vi "Teleop.vi"(10 "Match Info":T1={"Autonomous Elapsed Seconds"=0.0, "TeleOp Elapsed Seconds"=0.0, "Disabled Elapsed Seconds"=0.0, "Visited Autonomous"=FALSE, "Visited TeleOp"=FALSE, "Visited Disabled"=FALSE, "Autonomous Settings"={"Autonomous Style"=enum."Independent", "VI Refnum"=refnum}}, 11 "Call Context":T2) -> ()   [LabVIEW 2015]
doc: "This VI is called for each TeleOp packet received from the DS where the robot is not disabled. It is often used to read from the joysticks and update I/O or to update setpoints for timed control loops. It should complete and return within 20 milliseconds or it may miss DS packets."
uses:
  <vilib>/Rock Robotics/WPI/DriverStation/WPI_DriverStationDerivedRobotMode.ctl
  <vilib>/Rock Robotics/WPI/DriverStation/WPI_DriverStationMatch Info.ctl
  <vilib>/Rock Robotics/WPI/Utilities/WPI_GetSetVariantRefNum.vi
  <vilib>/Rock Robotics/Network Tables/NT Write Boolean Array.vi
  <vilib>/Rock Robotics/Network Tables/NT Write Numeric Array.vi
  <vilib>/Rock Robotics/WPI/RobotDrive/WPI_RobotDriveMecanumDrive_Cartesian.vi
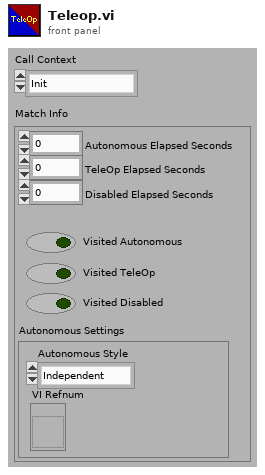
[diagram p1: front panel]
types:
  T1 = typedef "WPI_DriverStationMatch Info.ctl" = cluster{"Autonomous Elapsed Seconds":dbl, "TeleOp Elapsed Seconds":dbl, "Disabled Elapsed Seconds":dbl, "Visited Autonomous":bool, "Visited TeleOp":bool, "Visited Disabled":bool, "Autonomous Settings":cluster{"Autonomous Style":enum16{"Iterative", "Independent"}, "VI Refnum":refnum<vi>}}
  T2 = typedef "WPI_DriverStationDerivedRobotMode.ctl" = enum16{"Init", "Execute", "Stop"}
  T3 = typedef "WPI_JoystickDevRef.ctl" = cluster{"Device":T4}
  T4 = typedef "WPI_JoystickDeviceEnum.ctl" = enum16{"USB 0", "USB 1", "USB 2", "USB 3", "USB 4", "USB 5"}
  T5 = typedef "WPI_RobotDriveDevRef.ctl" = cluster{"DevStatus":errorcluster, "Motors[]":T6[], "Square Inputs":bool, "Max Output":dbl}
  T6 = typedef "WPI_MotorControlDeviceRef.ctl" = cluster{"DeviceStatus":errorcluster, "Type":T7, "PWM":cluster{"PWM Channel":T8, "DeadBand":T9}, "CAN":cluster{"Device Number":u8, "Control Mode":T10, "Semaphore":T11, "Max Vout":dbl, "TalonSRX Control Mode":T12}, "Invert":bool}
  T7 = typedef "WPI_MotorControlType.ctl" = enum16{"PWM", "CAN", "CANTalonSRX"}
  T8 = typedef "FPGA_DIOPWMChannel.ctl" = enum8{"PWM 0", "PWM 1", "PWM 2", "PWM 3", "PWM 4", "PWM 5", "PWM 6", "PWM 7", "PWM 8", "PWM 9", "PWM MXP 0", "PWM MXP 1", "PWM MXP 2", "PWM MXP 3", "PWM MXP 4", "PWM MXP 5", "PWM MXP 6", "PWM MXP 7", "PWM MXP 8", "PWM MXP 9", "Invalid"}
  T9 = typedef "WPI_PWMDeadband.ctl" = cluster{"Name":string, "maxPositivePwm":i32, "minPositivePwm":i32, "centerPwm":i32, "maxNegativePwm":i32, "minNegativePwm":i32, "angularRange":u16}
  T10 = typedef "WPI_CANJaguar_ControlMode.ctl" = enum8{"Percent VBus", "Current", "Speed", "Position", "Voltage"}
  T11 = typedef "Semaphore RefNum" = refnum<k1>
  T12 = typedef "WPI_CANTalonSRX_APIControlMode.ctl" = enum8{"Percent VBus", "Speed", "Position", "Slave", "Unchanged / Invalid", "Voltage Compensation", "Current", "Motion Profile"}
  T13 = typedef "WPI_GyroDevRef.ctl" = cluster{"DevStatus":errorcluster, "Analog Channel":T14, "Offset":dbl, "Gain (VoltsPerDegree/Second)":dbl, "Gyro Type":enum16{"Analog", "XRS450"}, "Handle":i32, "SPI Bus":T15, "Device Found":bool, "Sample Rate":dbl, "Calibrate On Open":bool}
  T14 = typedef "FPGA_AIChannel.ctl" = enum8{"AI 0", "AI 1", "AI 2", "AI 3", "AI MXP 0", "AI MXP 1", "AI MXP 2", "AI MXP 3", "Invalid"}
  T15 = typedef "spi_bus.ctl" = enum16{"SPI On-Board, CS0", "SPI On-Board, CS1", "SPI On-Board, CS2", "SPI On-Board, CS3", "SPI MXP", "Invalid"}
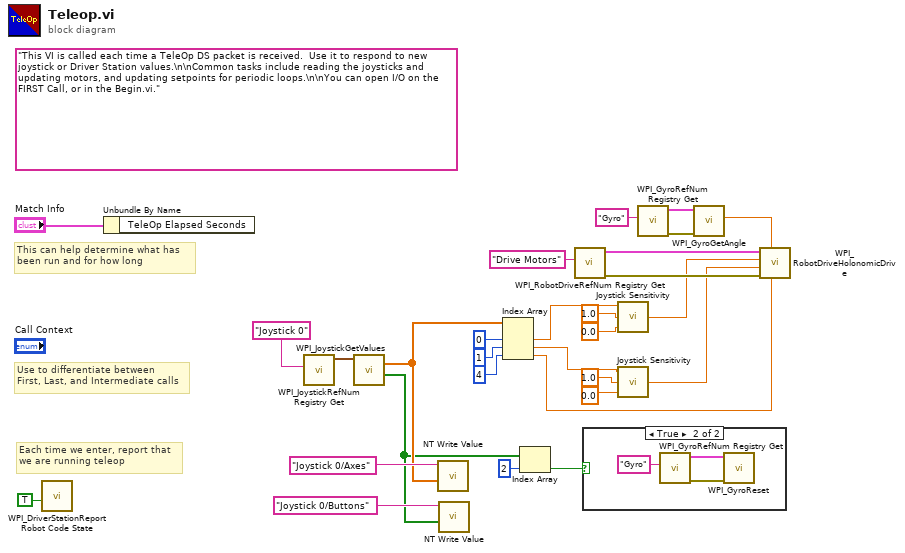
[diagram p0: block diagram]
diagram:
  (unwired) "This VI is called each time a TeleOp DS packet is received.  Use it to respond to new joystick or Driver Station values.\n\nCommon tasks include reading the joysticks and updating motors, and updating setpoints for periodic loops.\n\nYou can open I/O on the FIRST Call, or in the Begin.vi."
  # "Each time we enter, report that\nwe are running teleop"
  # "Use to differentiate between\nFirst, Last, and Intermediate calls"
  # "This can help determine what has\nbeen run and for how long"
  n1 = call <vilib>:"WPI_DriverStationReport Robot Code State.vi"("TeleOp"=TRUE ("Autonomous")) -> ()  [unwired: 10 in, 1 out]
  n2 = Unbundle By Name("Match Info") -> ()  [unwired: 1 out]
  n3 = call <vilib>:"WPI_JoystickRefNum Registry Get.vi"("refnum name"="Joystick 0") -> ("JoystickDevRef"=w24:T3)  [unwired: 1 in, 9 out]
  n4 = call <vilib>:"WPI_JoystickGetValues.vi"("JoystickDevRef"=w24) -> ("Buttons"=w7:bool[], "Axes"=w8:dbl[])  [unwired: 6 in, 3 out]
  n5 = call-poly <vilib>:"NT Write Value.vi"("Numeric Array"=w8, "Name"="Joystick 0/Axes") -> ()  [unwired: 9 in, 1 out]
  n6 = call-poly <vilib>:"NT Write Value.vi"("Boolean Array"=w7, "Name"="Joystick 0/Buttons") -> ()  [unwired: 9 in, 1 out]
  n7 = Index Array(array=w8, index #1=0 ("index"), index #2=1 ("index"), index #3=4 ("index")) -> (element #1=w11:dbl, element #2=w14:dbl, element #3=w1:dbl)
  n8 = Index Array(array=w7, index=2) -> (element=w5:bool)
  n9 = call <vilib>:"WPI_RobotDriveRefNum Registry Get.vi"("refnum name"="Drive Motors") -> ("error out"=w16:errorcluster, "RobotDriveDevRef"=w17:T5)  [unwired: 9 in]
  n10 = case shown="True" w5 {
    frame False {
    }
    frame True {
      n11 = call <vilib>:"WPI_GyroRefNum Registry Get.vi"("refnum name"="Gyro") -> ("error out"=w30:errorcluster, "GyroDevRef"=w31:T13)  [unwired: 9 in]
      n12 = call <vilib>:"WPI_GyroReset.vi"("error in"=w30, "GyroDevRef"=w31) -> ()  [unwired: 8 in, 2 out]
    }
  }
  n13 = call "Joystick Sensitivity.vi"("B"=0.0, "A"=1.0, "X"=w11) -> ("Y"=w3:dbl)
  n14 = call "Joystick Sensitivity.vi"("B"=0.0, "A"=1.0, "X"=w14) -> ("Y"=w2:dbl)
  n15 = call <vilib>:"WPI_GyroRefNum Registry Get.vi"("refnum name"="Gyro") -> ("error out"=w19:errorcluster, "GyroDevRef"=w18:T13)  [unwired: 9 in]
  n16 = call <vilib>:"WPI_GyroGetAngle.vi"("error in"=w19, "GyroDevRef"=w18) -> ("Angle"=w4:dbl)  [unwired: 5 in, 4 out]
  n17 = call-poly <vilib>:"WPI_RobotDriveHolonomicDrive.vi"("Rotation"=w1, "Gyro Angle"=w4, "error in (no error)"=w16, "Y"=w2, "X"=w3, "RobotDriveDevRef"=w17) -> ()  [unwired: 3 in, 3 out]
